vi "Check File.vi"(6 "Search String":string, 7 "Offset String":string, 9 "List of Key File":path, 11 "Operative File":path) -> (0 "Line of Error":i32, 2 "Bad String":string, 3 "Any Errors":bool, 5 "File Path Out":path)   [LabVIEW 2017]
uses:
  <vilib>/Utility/file.llb/Read Delimited Spreadsheet (string).vi
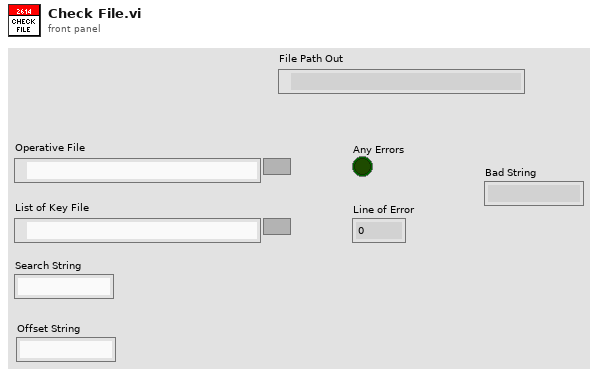
[diagram p1: front panel]
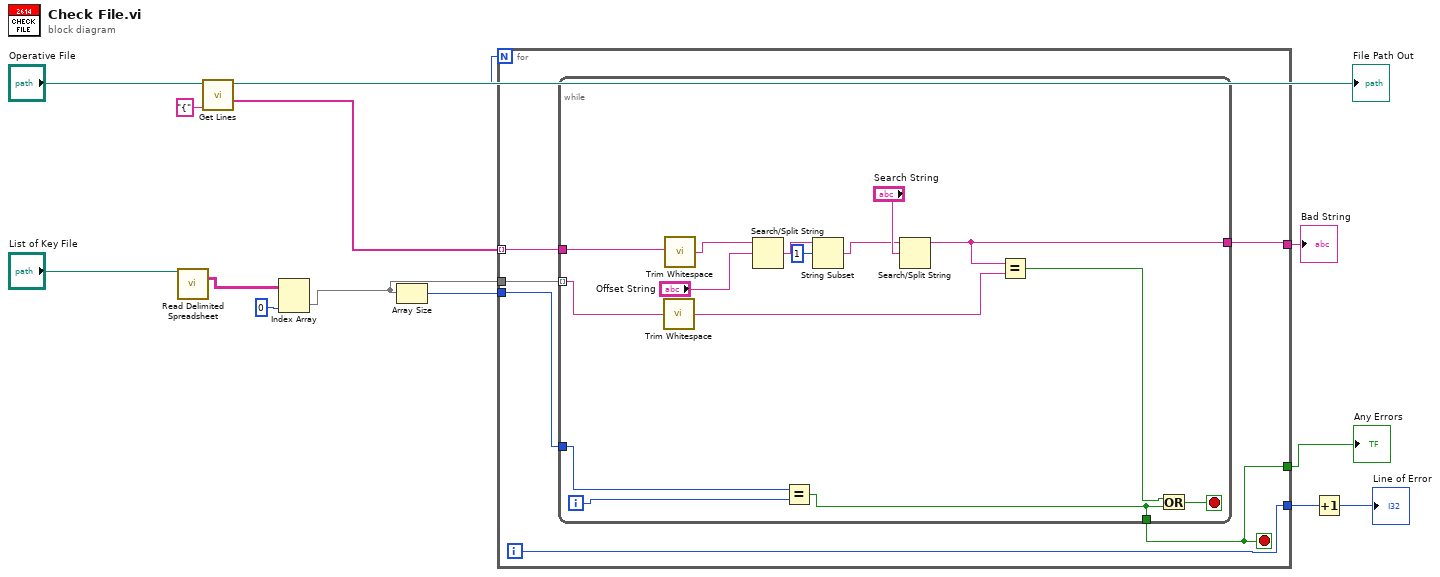
[diagram p0: block diagram]
diagram:
  n1 = call-poly <vilib>:"Read Delimited Spreadsheet.vi"("file path (dialog if empty)"="List of Key File") -> ("all rows"=w9:string[][])  [unwired: 9 in, 5 out]
  n2 = call "Get Lines.vi"("Start of Commands"="{", "Auto File"="Operative File") -> ("Lines"=w3:string[], "Lines of File"=w2:i32)  [unwired: 6 in]
  n3 = Index Array(array=w9, index (col)=0 ("disabled index (col)")) -> (element=w8:string[])  [unwired: 1 in]
  n4 = Array Size(array=w8) -> (size(s)=w13:i32)
  n5 = for {
    N: w2 -> [_]
    tunnel: w3 -> [w18] mode=indexing
    tunnel: w8 -> [w19]
    tunnel: w13 -> [w17]
    tunnel: [w16] -> w5
    tunnel: [w15] -> w12
    tunnel: [w14] -> w6
    i -> [w15]
    stop <- w16 stop-if-true
    n6 = while {
      tunnel: w19 -> [w34] mode=indexing
      tunnel: w18 -> [w33]
      tunnel: w17 -> [w32]
      tunnel: [w28] -> w16
      tunnel: [w25] -> w14
      i -> [w31]
      stop <- w30 stop-if-true
      n7 = call <vilib>:"Trim Whitespace.vi"("string"=w34) -> ("trimmed string"=w26:string)  [unwired: 1 in]
      n8 = call <vilib>:"Trim Whitespace.vi"("string"=w33) -> ("trimmed string"=w23:string)  [unwired: 1 in]
      n9 = Search/Split String(string=w23, search string/char (-)="Offset String") -> (match + rest of string=w21:string)  [unwired: 1 in, 2 out]
      n10 = Equal?(x=w32, y=w31) -> (x = y?=w28:bool)
      n11 = String Subset(string=w21, offset (0)=1) -> (substring=w22:string)  [unwired: 1 in]
      n12 = Search/Split String(string=w22, search string/char (-)="Search String") -> (substring before match=w25:string)  [unwired: 1 in, 2 out]
      n13 = Equal?(x=w25, y=w26) -> (x = y?=w29:bool)
      n14 = Or(x=w29, y=w28) -> (x .or. y?=w30:bool)
    }
  }
  "Any Errors" <- w5
  "Bad String" <- w6
  n15 = Increment(x=w12) -> (x+1=→"Line of Error":i32)
  "File Path Out" <- "Operative File"
